vi "Dashboard Main.vi"() -> ()   [LabVIEW 2015]
uses:
  <vilib>/Utility/miscctls.llb/LVRowAndColumnTypeDef.ctl
  <vilib>/event_ctls.llb/eventvkey.ctl
  <vilib>/Rock Robotics/WPI/Dashboard/WPI_DashboardLogging Global.vi
  <vilib>/Rock Robotics/Network Tables/NT Read Numeric Array.vi
  <vilib>/Rock Robotics/Network Tables/NT Write String Array.vi
  <vilib>/Utility/config.llb/Write Key (String).vi
  <vilib>/Utility/config.llb/Write Key (I32).vi
  <vilib>/Utility/config.llb/NI_LVConfig.lvlib
panel:
  in  "TCP":refnum<k5>
  in  "Rec Mode":enum32{"Stop", "Record", "Playback"}(radio)
  in  "Vision":u16(ring) items=["Camera Off", "USB Camera SW", "USB Camera HW", "IP Camera"]
  out "Camera IP":string
  out "Image Message":string="Timeout in Camera Communications"
  in  "Dashboard Tab":T1(tab)
  in  "Select Auto":string(combo)
  out "NT Connection":bool
  in  "Camera Settings":T2={"Frame Rate"=30, "Compression"=30, "Size"=1} {"Frame Rate" scale=1.0..30.0; "Size" items=["640x480", "320x240", "160x120"]}
  out "MotorChart R":cluster{"Numeric":dbl, "Numeric":dbl}(graph)
  out "MotorChart L":T3(graph)
  out "MotorSliders R":cluster{"MotorSlide1":dbl, "MotorSlide2":dbl} {"MotorSlide2" scale=-1.0..1.0 scale format="%#_2e"; "MotorSlide1" scale=-1.0..1.0 scale format="%#_2e"}
  out "MotorSliders L":T4 {"MotorSlide4 2" scale=0.0..14.0 scale format="%#_2e"; "MotorSlide2" scale=-1.0..1.0 scale format="%#_2e"; "MotorSlide1" scale=-1.0..1.0 scale format="%#_2e"}
  out "JS1 Z":dbl(slide) scale=-1.0..1.0 scale format="%#_2e"
  out "JS1 Graph":cluster{"X":dbl, "Y":dbl}[](graph)
  out "JS1 Buttons":T5
  out "JS2 Z":dbl(slide) scale=-1.0..1.0 scale format="%#_2e"
  out "JS2 Graph":cluster{"X":dbl, "Y":dbl}[](graph)
  out "JS2 Buttons":T5
  out "Mode":T6(ring)=enum."Auto Disabled"
  in  "DB Camera Config":bool
  out "fps":dbl format="%#.1g"
  out "Mbps":dbl format="%#.1g"
  out "Mbps LED":bool
  in  "DB/String 9":string
  in  "DB/String 8":string
  in  "DB/String 7":string
  in  "DB/String 6":string
  in  "DB/String 5":string
  in  "DB/String 4":string
  in  "DB/String 3":string
  in  "DB/String 2":string
  in  "DB/String 1":string
  in  "DB/String 0":string
  in  "DB/Slider 0":dbl(slide) scale=0.0..5.0
  in  "DB/Slider 1":dbl(slide) scale=0.0..5.0
  in  "DB/Slider 2":dbl(slide) scale=0.0..5.0
  in  "DB/Slider 3":dbl(slide) scale=0.0..5.0
  out "DB/LED 3":bool
  out "DB/LED 2":bool
  out "DB/LED 1":bool
  out "DB/LED 0":bool
  in  "DB/Button 3":bool
  in  "DB/Button 2":bool
  in  "DB/Button 1":bool
  in  "DB/Button 0":bool caption="New Name"
  out "IMU AHRS":dbl[](array[numeric])
  out "CAN Current Values":dbl[](array[numeric])
  out "Arm Angle":dbl
  out "Right LIDAR":dbl
  out "Left LIDAR":dbl
  out "Right Encoder":dbl
  out "Left Encoder":dbl
  out "Ultrasonic Sensors":dbl[](array[numeric])
  out "SPI Gyro":dbl
  out "IMU AHRS Delta":dbl[](array[numeric])
  out "Goal Position":string
  out "appended array":string[](array[string])
  out "Position":i32
  out "Numeric":i32
  in  "Test Slider":dbl(slide) scale=0.0..100.0 scale format="%#_3g"
  in  "On/Off":bool caption="Solenoid"
  in  "Test Name":u16(ring) items=["Select the test to run..."]
  in  "Test Tree":string(tree)
  in  "Motor":cluster{"Value":dbl, "Enable":bool} {"Value" scale=-1.0..1.0 scale format="%#_3g"}
  out "Progress":T7 {"Test Progress" scale=0.0..100.0}
  in  "Rev/Fwd":cluster{"Forward":bool, "Reverse":bool}
  in  "Test Ring":u16(ring) items=["Monochrome", "Color"]
  out "Cmd Status":string
  in  "Execute Command":bool
  in  "Command Params":string[][](table)
  in  "Command Selection":i32(listbox)
  in  "Defence 5":bool
  in  "Defence 4":bool
  in  "Defence 3":bool
  in  "Defence 2":bool
  in  "Defence 1":bool
  in  "Defense 5":u16(ring)=8 items=["", "Portcullis", "Chili Fries", "Moat", "Ramparts", "Drawbridge", "Sally Port", "Rock Wall", "Rough Terrain"]
  in  "Defense 2":u16(ring)=8 items=["", "Portcullis", "Chili Fries", "Moat", "Ramparts", "Drawbridge", "Sally Port", "Rock Wall", "Rough Terrain"]
  in  "Defense 3":u16(ring)=8 items=["", "Portcullis", "Chili Fries", "Moat", "Ramparts", "Drawbridge", "Sally Port", "Rock Wall", "Rough Terrain"]
  in  "Defense 4":u16(ring)=8 items=["", "Portcullis", "Chili Fries", "Moat", "Ramparts", "Drawbridge", "Sally Port", "Rock Wall", "Rough Terrain"]
  in  "Defense 1":string="Low Bar"
  out "Robot":bool
  in  "Goal Position 3":u16(ring)=8 items=["", "Left", "Center", "Right"]
  in  "Goal Position 2":u16(ring)=8 items=["", "High", "Low"]
  in  "CheckList":i32(listbox)
  out "Tree":string(tree)
  out "Camera Image":T8(plugin-control)
  out "Background":bool
  # "Left"
  # "Front"
  # "Right"
  # "Battery"
  # "Pitch"
  # "Roll"
  # "Yaw"
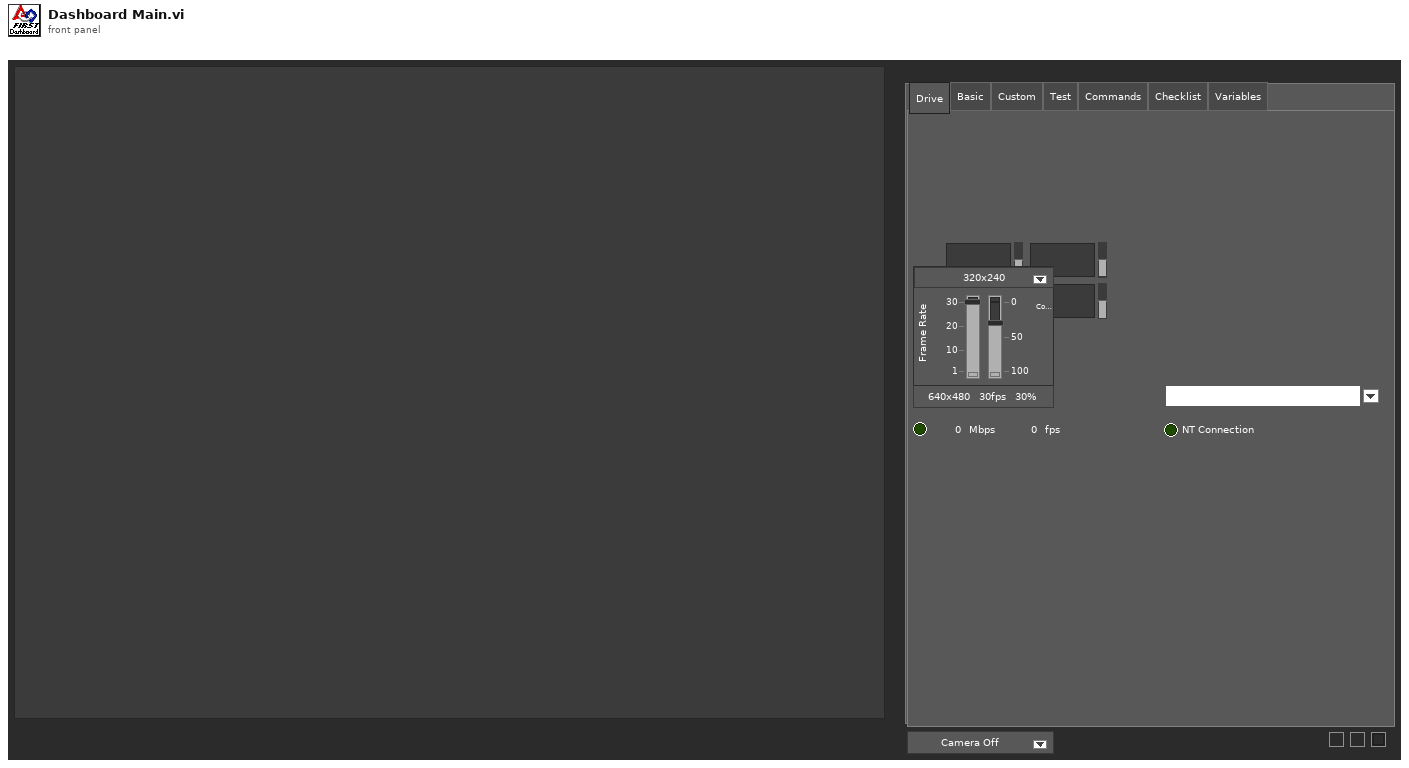
[diagram p1: front panel]
types:
  T1 = enum32{"Drive", "Basic", "Custom", "Test", "Commands", "Checklist", "Variables"}
  T2 = cluster{"Frame Rate":i32, "Compression":i32, "Size":u16}
  T3 = cluster{"Numeric":dbl, "Numeric":dbl, "Battery V":dbl}
  T4 = cluster{"MotorSlide1":dbl, "MotorSlide2":dbl, "MotorSlide4 2":dbl}
  T5 = cluster{bool, bool, bool, bool, bool, bool, bool, bool, bool, bool, bool, bool}
  T6 = enum8{"Tele-Op Disabled", "Tele-Op Enabled", "Auto Disabled", "Auto Enabled", "Test Disabled", "Test Enabled", "Disconnected", "No Code", "E-Stop"}
  T7 = cluster{"Test Progress":u8, "Test Progress Text":string}
  T8 = typedef "IMAQ Image.ctl" = refnum<image>
  T9 = cluster{"IDs":cluster{"RPC field ID":u16, "Unique ID":u16}, "String":string}
  T10 = enum32{"Drive", "Basic", "Custom", "Test", "Checklist", "Variables"}
  T11 = typedef "Image Type" = u32
  T12 = cluster{"Camera Image":refnum<vi>, "Dashboard Tab":refnum<vi>, "Background":refnum<vi>, "Vision":refnum<vi>, "Rec Mode":refnum<vi>, "Test Slider":refnum<vi>, "On/Off ":refnum<vi>, "Test Ring":refnum<vi>, "Rev/Fwd":refnum<vi>, "Test Name":refnum<vi>, "Motor":refnum<vi>, "Progress":refnum<vi>, "CheckList":refnum<vi>, "Tree":refnum<vi>, "Test Tree":refnum<vi>, "Command Params":refnum<vi>, "Command Selection":refnum<vi>, "Execute Command":refnum<vi>, "Cmd Status":refnum<vi>}
  T13 = cluster{"Error Strings":string, "Disable Counts":cluster{u16, u16}, "Rail Faults":cluster{u16, u16, u16}, "Robot IP":string, "DB Mode":u8, "Event Info":cluster{"Name":string, "Type":u8, "Number":u16, "Replay":u8}, "Camera Addr":string}
  T14 = cluster{"Storage":cluster{"Disk Free":u64, "RAM Block":u32, "RAM free":u32}, "CPU Utilization":cluster{"CPU % ISR":sgl, "CPU % Time Crit":sgl, "CPU % Timed Str":sgl, "CPU % High":sgl, "CPU % Above":sgl, "CPU % Normal":sgl, "CPU % Low":sgl}, "CAN":cluster{"% Bus Utilization":sgl, "Bus Off Cnt":u32, "TX_FIFO Full Cnt":u32, "Receive Error Cnt":u8, "Transmit Error Cnt":u8}, "HID":cluster{"HID Outputs":u32, "Rumble Low":u16, "Rumble High":u16}[]}
  T15 = cluster{"Status bits":cluster{"Test Mode":bool, "Autonomous":bool, "Enabled":bool, "Code Start":bool, "Brownout":bool, "Reserved 2":bool, "Reserved 3":bool, "E-Stop":bool}, "Code Trace":cluster{"Disabled":bool, "TeleOp":bool, "Auto":bool, "Test":bool}, "Controller Type":enum16{"unknown", "cRIO", "roboRio"}, "Code?":enum16{"unknown", "noCode", "code"}, "Battery V":dbl}
  T16 = cluster{"Control Bits":cluster{"TestMode":bool, "Autonomous":bool, "Enabled":bool, "FMS Present":bool, bool, bool, bool, "E-Stop":bool}, "Team Station ":u8, "Countdown":sgl, "Joystick Values":cluster{"Axes":dbl[], "Buttons":bool[], "POVs":i16[]}[]}
  T17 = cluster{"Axes":dbl[], "Buttons":bool[], "POVs":i16[]}[]
  T18 = cluster{"Axes":dbl[], "Buttons":bool[], "POVs":i16[]}
  T19 = cluster{"Buttons[0]":bool, "Buttons[1]":bool, "Buttons[2]":bool, "Buttons[3]":bool, "Buttons[4]":bool, "Buttons[5]":bool, "Buttons[6]":bool, "Buttons[7]":bool, "Buttons[8]":bool, "Buttons[9]":bool, "Buttons[10]":bool, "Buttons[11]":bool}
  T20 = typedef "NI_LVConfig.lvlib/Config Data RefNum.ctl" = refnum<k1>
  T21 = cluster{"Operation":enum16{"Update", "Clear"}, "Color Box":u32}[]
  T22 = typedef "eventvkey.ctl" = enum16{"ASCII", "Enter", "Return", "Shift", "Ctrl", "Alt", "Cmd", "Opt", "Caps", "NumLock", "Clear", "Break", "Up", "Down", "Left", "Right", "Insert", "Delete", "Home", "End", "PageUp", "PageDown", "Escape", "Help", "Pause", "ScrollLock", "F1", "F2", "F3", "F4", "F5", "F6", "F7", "F8", "F9", "F10", "F11", "F12", "F13", "F14", "F15", "F16", "F17", "F18", "F19", "F20", "F21", "F22", "F23", "F24", "Play", "VolumeUp", "VolumeDown", "Mute", "Two Byte Char"}
  T23 = cluster{"Image Size":bool, "Image Type":bool, "Pixel Value":bool, "ROI Information":bool, "Zoom Factor":bool}
  T24 = enum8{"Enabled", "Disabled", "Disabled and Grayed Out"}
  T25 = cluster{"Operation":enum16{"Update", "Clear"}, "Color Box":u32}
  T26 = typedef "LVRowAndColumnTypeDef.ctl" = cluster{"Row":i32, "Column":i32}
  T27 = cluster{"Shift":bool, "Ctrl":bool, "Alt":bool, "Cmd":bool, "Opt":bool}
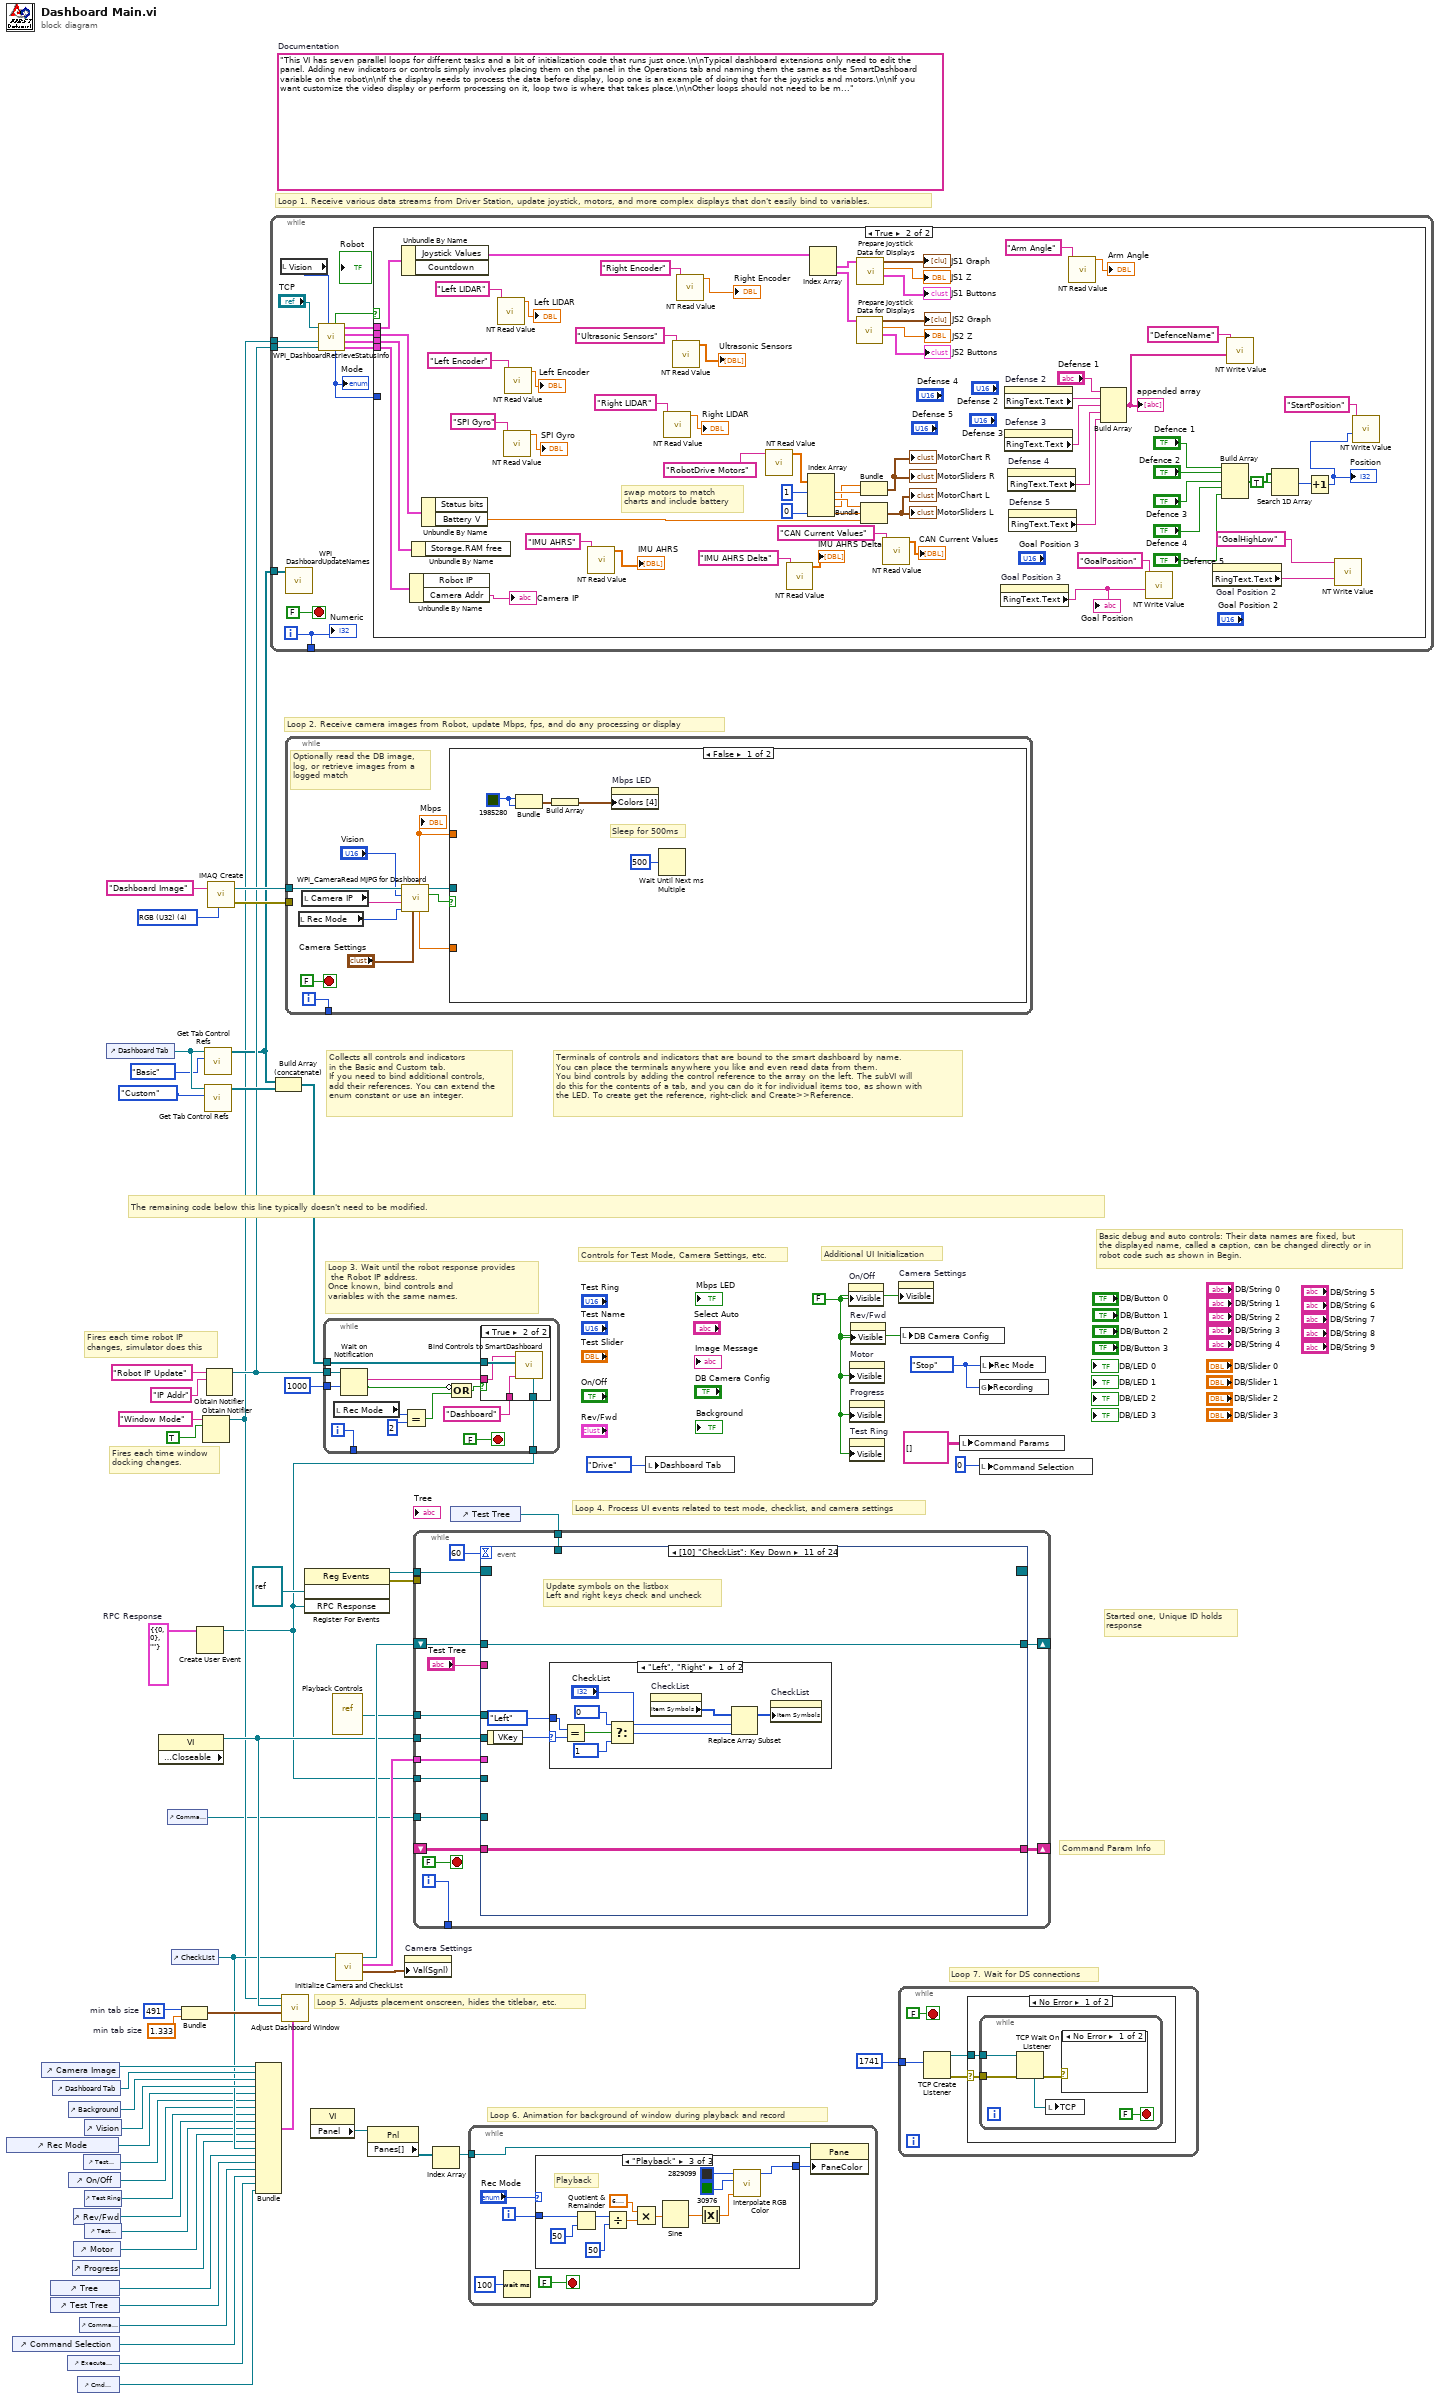
[diagram p0: block diagram]
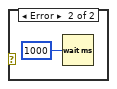
[diagram p2: hidden frame]
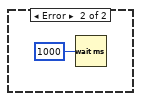
[diagram p3: hidden frame]
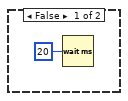
[diagram p4: hidden frame]
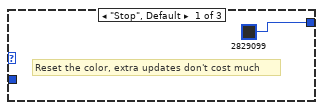
[diagram p5: hidden frame]
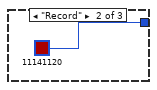
[diagram p6: hidden frame]
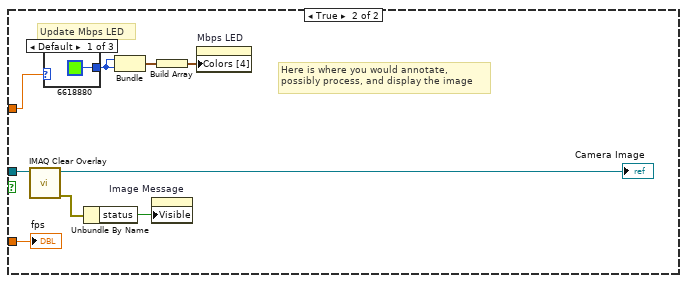
[diagram p8: hidden frame]
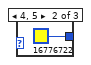
[diagram p9: hidden frame]
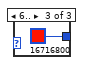
[diagram p10: hidden frame]
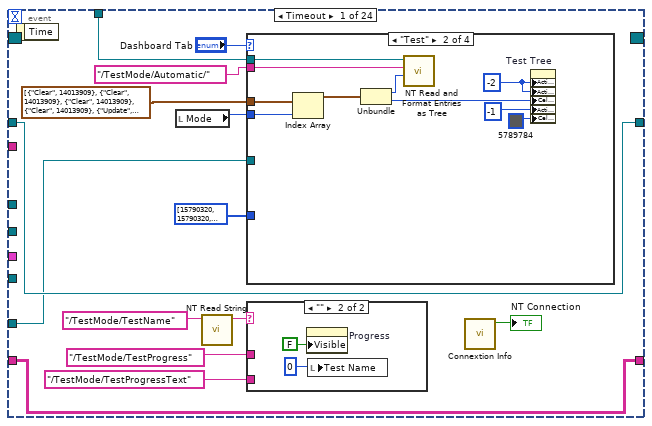
[diagram p11: hidden frame]
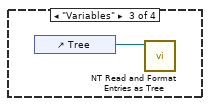
[diagram p13: hidden frame]
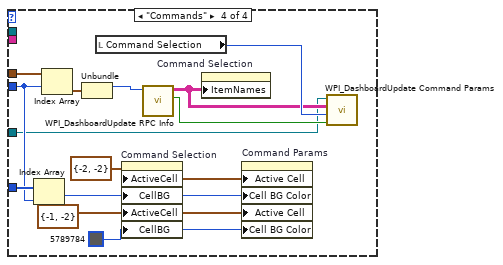
[diagram p14: hidden frame]
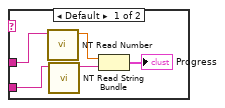
[diagram p15: hidden frame]
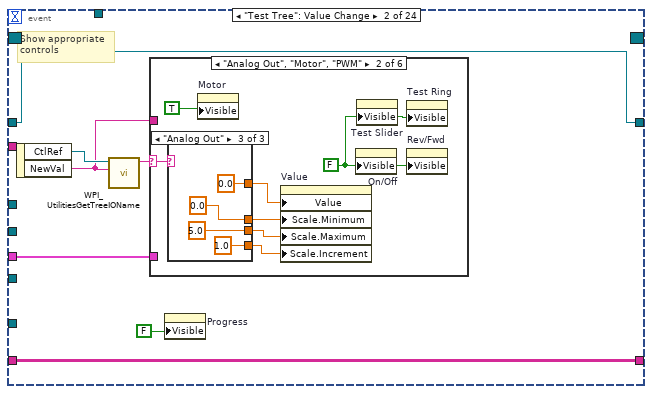
[diagram p16: hidden frame]
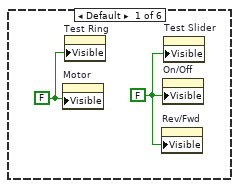
[diagram p17: hidden frame]
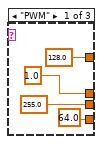
[diagram p18: hidden frame]
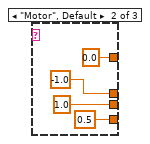
[diagram p19: hidden frame]
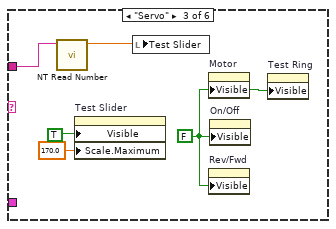
[diagram p20: hidden frame]
diagram:
  w7 = T9 {"IDs"={"RPC field ID"=0, "Unique ID"=0}, "String"=""}  # RPC Response
  w33 = 491  # min tab size
  w32 = 1.333  # min tab size
  w41 = enum32{"Stop", "Record", "Playback"}."Stop" ("Rec Mode")
  w15 = FALSE ("Visible")
  (unwired) "This VI has seven parallel loops for different tasks and a bit of initialization code that runs just once.\n\nTypical dashboard extensions only need to edit the panel. Adding new indicators or controls simply involves placing them on the panel in the Operations tab and naming them the same as the SmartDashboard variable on the robot\n\nIf the display needs to process the data before display, loop one is an example of doing that for the joysticks and motors.\n\nIf you want customize the video display or perform processing on it, loop two is where that takes place.\n\nOther loops should not need to be modified. They are pretty standard, and document the task they perform."  # Documentation
  w61 = T11 4 items=["Grayscale (U8)", "Grayscale (I16)", "Grayscale (SGL)", "Complex (CSG)", "RGB (U32)", "HSL (U32)", "RGB (U64)"] ("Image Type")
  # "Command Param Info"
  # "Started one, Unique ID holds\nresponse"
  # "Loop 7. Wait for DS connections"
  # "Basic debug and auto controls: Their data names are fixed, but\nthe displayed name, called a caption, can be changed directly or in\nrobot code such as shown in Begin."
  # "Controls for Test Mode, Camera Settings, etc."
  # "Additional UI Initialization"
  # "Loop 6. Animation for background of window during playback and record"
  # "Fires each time robot IP\nchanges, simulator does this"
  # "Fires each time window\ndocking changes."
  # "Collects all controls and indicators\nin the Basic and Custom tab.\nIf you need to bind additional controls,\nadd their references. You can extend the\nenum constant or use an integer."
  # "The remaining code below this line typically doesn't need to be modified."
  # "Loop 4. Process UI events related to test mode, checklist, and camera settings"
  # "Terminals of controls and indicators that are bound to the smart dashboard by name.\nYou can place the terminals anywhere you like and even read data from them.\nYou bind controls by adding the control reference to the array on the left. The subVI will\ndo this for the contents of a tab, and you can do it for individual items too, as shown with\nthe LED. To create get the reference, right-click and Create>>Reference."
  # "Loop 3. Wait until the robot response provides\n the Robot IP address.\nOnce known, bind controls and\nvariables with the same names."
  # "Loop 5. Adjusts placement onscreen, hides the titlebar, etc."
  # "Loop 1. Receive various data streams from Driver Station, update joystick, motors, and more complex displays that don't easily bind to variables."
  # "Loop 2. Receive camera images from Robot, update Mbps, fps, and do any processing or display"
  n1 = control-ref of="Rec Mode"() -> (w21:refnum<vi>)
  n2 = control-ref of="Command Selection"() -> (w6:refnum<vi>)
  n3 = control-ref of="Camera Image"() -> (w36:refnum<vi>)
  n4 = control-ref of="Tree"() -> (w25:refnum<vi>)
  n5 = control-ref of="Test Tree"() -> (w24:refnum<vi>)
  n6 = control-ref of="Dashboard Tab"() -> (w35:refnum<vi>)
  n7 = control-ref of="Execute Command"() -> (w8:refnum<vi>)
  n8 = control-ref of="Background"() -> (w30:refnum<vi>)
  n9 = control-ref of="On/Off"() -> (w19:refnum<vi>)
  n10 = control-ref of="Progress"() -> (w16:refnum<vi>)
  n11 = control-ref of="Rev/Fwd"() -> (w17:refnum<vi>)
  n12 = control-ref of="Motor"() -> (w22:refnum<vi>)
  n13 = control-ref of="Cmd Status"() -> (w2:refnum<vi>)
  n14 = control-ref of="Command Params"() -> (w9:refnum<vi>)
  n15 = control-ref of="Test Slider"() -> (w20:refnum<vi>)
  n16 = control-ref of="Vision"() -> (w34:refnum<vi>)
  n17 = control-ref of="Test Ring"() -> (w18:refnum<vi>)
  n18 = control-ref of="Test Name"() -> (w23:refnum<vi>)
  n19 = control-ref of="Dashboard Tab"() -> (w39:refnum<vi>)
  n20 = property class="VI" props=["Front Panel.Closeable"]() -> (reference out=w40:refnum<vi>)  [unwired: 2 in, 2 out]
  n21 = control-ref of="Command Params"() -> (w1:refnum<vi>)
  n22 = control-ref of="CheckList"() -> (w26:refnum<vi>)
  n23 = Bundle("min tab size"=w33, "min tab size"=w32) -> (w31:cluster{"min tab size":i32, "min tab size":dbl})  [unwired: 1 in]
  n24 = Create User Event(user event datatype=w7) -> (user event=w3:refnum<user-event>)  [unwired: 1 in, 1 out]
  n25 = Obtain Notifier(name (unnamed)="Window Mode", notification data type=TRUE) -> (notifier out=w12:refnum<notifier>)  [unwired: 2 in, 2 out]
  n26 = call <vilib>:"Get Tab Control Refs.vi"("Page Index"=T10."Basic" ("Dashboard Tab"), "TabControl in"=w39) -> ("ControlsOnPage"=w13:refnum<vi>[])  [unwired: 9 in]
  n27 = call <vilib>:"Get Tab Control Refs.vi"("Page Index"=T10."Custom" ("Dashboard Tab"), "TabControl in"=w39) -> ("ControlsOnPage"=w38:refnum<vi>[])  [unwired: 9 in]
  n28 = Obtain Notifier(name (unnamed)="Robot IP Update", notification data type="IP Addr" ("name (unnamed)")) -> (notifier out=w14:refnum<notifier>)  [unwired: 2 in, 2 out]
  n29 = call "IMAQ Create"("Image Name"="Dashboard Image", "Image Type"=w61) -> ("New Image"=w59:T8, "error out"=w58:errorcluster)  [unwired: 2 in, 1 out]
  n30 = Bundle("Camera Image"=w36, "Dashboard Tab"=w35, "Background"=w30, "Vision"=w34, "Rec Mode"=w21, "Test Slider"=w20, "On/Off"=w19, "Test Ring"=w18, "Rev/Fwd"=w17, "Test Name"=w23, "Motor"=w22, "Progress"=w16, "CheckList"=w26, "Tree"=w25, "Test Tree"=w24, "Command Params"=w9, "Command Selection"=w6, "Execute Command"=w8, "Cmd Status"=w2) -> (w27:T12)  [unwired: 1 in]
  n31 = while {
    tunnel: [w73] -> _
    tunnel: w14 -> [w67]
    tunnel: w13 -> [w66]
    tunnel: w12 -> [w62]
    i -> [w73]
    stop <- FALSE stop-if-true
    n32 = local read "Vision"() -> (w64:u16)
    n33 = call <vilib>:"WPI_DashboardUpdateNames.vi"("Controls on Tab"=w66) -> ()  [unwired: 11 in]
    n34 = call <vilib>:"WPI_DashboardRetrieveStatusInfo.vi"("Vision"=w64, "Binding Refnum"=w67, "Window Mode Notifier"=w62, "TCP Cnx"="TCP") -> ("Power and Errors"=w68:T13, "Robot Metrics"=w71:T14, "Status Info"=w72:T15, "Control Info"=w69:T16, "Robot Mode"=w65:T6, "Process?"=w70:bool)  [unwired: 2 in]
    "Mode" <- w65
    n35 = case shown="True" w70 {
      tunnel: w72 -> [_ w141]
      tunnel: w71 -> [_ w140]
      tunnel: w69 -> [_ w139]
      tunnel: w68 -> [_ w138]
      tunnel: w65 -> [_ _]
      frame False {
        n36 = Wait (ms)(milliseconds to wait=u32 20) -> ()  [unwired: 1 out]
      }
      frame True {
        # "swap motors to match\ncharts and include battery"
        n37 = Unbundle By Name(w139) -> ("Joystick Values"=w128:T17)  [unwired: 1 out]
        n38 = Unbundle By Name(w138) -> ("Camera Addr"=→"Camera IP":string)  [unwired: 1 out]
        n39 = Unbundle By Name(w140) -> ()  [unwired: 1 out]
        n40 = Unbundle By Name(w141) -> ("Battery V"=w129:dbl)  [unwired: 1 out]
        n41 = call-poly <vilib>:"NT Read Value.vi"("Name"="Left LIDAR") -> ("Numeric"=→"Left LIDAR":dbl)  [unwired: 9 in, 1 out]
        n42 = call-poly <vilib>:"NT Read Value.vi"("Name"="SPI Gyro") -> ("Numeric"=→"SPI Gyro":dbl)  [unwired: 9 in, 1 out]
        n43 = call-poly <vilib>:"NT Read Value.vi"("Name"="Left Encoder") -> ("Numeric"=→"Left Encoder":dbl)  [unwired: 9 in, 1 out]
        n44 = call-poly <vilib>:"NT Read Value.vi"("Name"="IMU AHRS") -> ("Numeric Array"=→"IMU AHRS":dbl[])  [unwired: 9 in, 1 out]
        n45 = call-poly <vilib>:"NT Read Value.vi"("Name"="Right LIDAR") -> ("Numeric"=→"Right LIDAR":dbl)  [unwired: 9 in, 1 out]
        n46 = call-poly <vilib>:"NT Read Value.vi"("Name"="Ultrasonic Sensors") -> ("Numeric Array"=→"Ultrasonic Sensors":dbl[])  [unwired: 9 in, 1 out]
        n47 = call-poly <vilib>:"NT Read Value.vi"("Name"="Right Encoder") -> ("Numeric"=→"Right Encoder":dbl)  [unwired: 9 in, 1 out]
        n48 = call-poly <vilib>:"NT Read Value.vi"("Name"="RobotDrive Motors") -> ("Numeric Array"=w117:dbl[])  [unwired: 9 in, 1 out]
        n49 = call-poly <vilib>:"NT Read Value.vi"("Name"="IMU AHRS Delta") -> ("Numeric Array"=→"IMU AHRS Delta":dbl[])  [unwired: 9 in, 1 out]
        n50 = Index Array(array=w117, index #1=1, index #4=0) -> (element #1=w133:dbl, element #2=w134:dbl, element #3=w132:dbl, element #4=w137:dbl)  [unwired: 2 in]
        n51 = Index Array(array=w128) -> (element #1=w127:T18, element #2=w122:T18)  [unwired: 2 in]
        n52 = call "Prepare Joystick Data for Displays.vi"("Joystick Values"=w122) -> ("Buttons"=→"JS2 Buttons":T19, "Z Axis"=→"JS2 Z":dbl, "Cartesian Data"=→"JS2 Graph":cluster{"X axis":dbl, "X axis":dbl}[])  [unwired: 8 in]
        n53 = call "Prepare Joystick Data for Displays.vi"("Joystick Values"=w127) -> ("Buttons"=→"JS1 Buttons":T19, "Z Axis"=→"JS1 Z":dbl, "Cartesian Data"=→"JS1 Graph":cluster{"X axis":dbl, "X axis":dbl}[])  [unwired: 8 in]
        n54 = Bundle("Numeric"=w132, "Numeric"=w133) -> (→"MotorChart R" →"MotorSliders R":cluster{"Numeric":dbl, "Numeric":dbl})  [unwired: 1 in]
        n55 = Bundle("Numeric"=w134, "Numeric"=w137, "Battery V"=w129) -> (→"MotorChart L" →"MotorSliders L":T3)  [unwired: 1 in]
        n56 = call-poly <vilib>:"NT Read Value.vi"("Name"="CAN Current Values") -> ("Numeric Array"=→"CAN Current Values":dbl[])  [unwired: 9 in, 1 out]
        n57 = property on="Goal Position 3" class="Ring (strict)"() -> ("RingText.Text"=w88:string)  [unwired: 2 in, 2 out]
        "Goal Position" <- w88
        n58 = property on="Defense 2" class="Ring (strict)"() -> ("RingText.Text"=w95:string)  [unwired: 2 in, 2 out]
        n59 = property on="Defense 3" class="Ring (strict)"() -> ("RingText.Text"=w94:string)  [unwired: 2 in, 2 out]
        n60 = property on="Defense 4" class="Ring (strict)"() -> ("RingText.Text"=w93:string)  [unwired: 2 in, 2 out]
        n61 = property on="Defense 5" class="Ring (strict)"() -> ("RingText.Text"=w92:string)  [unwired: 2 in, 2 out]
        n62 = call-poly <vilib>:"NT Read Value.vi"("Name"="Arm Angle") -> ("Numeric"=→"Arm Angle":dbl)  [unwired: 9 in, 1 out]
        n63 = Build Array("Defense 1", w95, w94, w93, w92) -> (w90:string[])
        "appended array" <- w90
        n64 = call-poly <vilib>:"NT Write Value.vi"("String"=w88, "Name"="GoalPosition") -> ()  [unwired: 9 in, 1 out]
        n65 = property on="Goal Position 2" class="Ring (strict)"() -> ("RingText.Text"=w76:string)  [unwired: 2 in, 2 out]
        n66 = Build Array("Defence 1", "Defence 2", "Defence 3", "Defence 4", "Defence 5") -> (w85:bool[])
        n67 = call-poly <vilib>:"NT Write Value.vi"("String Array"=w90, "Name"="DefenceName") -> ()  [unwired: 9 in, 1 out]
        n68 = Search 1D Array(1D array=w85, element=TRUE) -> (index of element=w87:i32)  [unwired: 1 in]
        n69 = Increment(x=w87) -> (x+1=w78:i32)
        "Position" <- w78
        n70 = call-poly <vilib>:"NT Write Value.vi"("String"=w76, "Name"="GoalHighLow") -> ()  [unwired: 9 in, 1 out]
        n71 = call-poly <vilib>:"NT Write Value.vi"("Numeric"=w78, "Name"="StartPosition") -> ()  [unwired: 9 in, 1 out]
      }
    }
    "Numeric" <- w73
  }
  n72 = Build Array (concatenate)(w13, w38) -> (w37:refnum<vi>[])
  n73 = call "Adjust Dashboard Window.vi"("Sizing Refnums"=w27, "Size Constraints"=w31, "VI"=w40, "WIn Mode"=w12) -> ()  [unwired: 8 in]
  n74 = while {
    tunnel: w59 -> [w150]
    tunnel: w58 -> [_]
    tunnel: [w151] -> _
    i -> [w151]
    stop <- FALSE stop-if-true
    # "Optionally read the DB image,\nlog, or retrieve images from a\nlogged match"
    n75 = local read "Rec Mode"() -> (w145:enum32{"Stop", "Record", "Playback"})
    n76 = local read "Camera IP"() -> (w143:string)
    n77 = call <vilib>:"WPI_CameraRead MJPG for Dashboard.vi"("Camera Settings"="Camera Settings", "Rec Mode"=w145, "Camera IP"=w143, "Camera Mode"="Vision", "Refnum in"=w150) -> ("Active"=w148:bool, "Refnum out"=w149:T8, "FPS"=w147:dbl, "Bandwidth (Mbps)"=w142:dbl)  [unwired: 3 in]
    "Mbps" <- w142
    n78 = case shown="False" w148 {
      tunnel: w149 -> [_ w160]
      tunnel: w142 -> [_ w159]
      tunnel: w147 -> [_ w157]
      frame False {
        w153 = u32 1985280 ("Color Box")
        # "Sleep for 500ms"
        n79 = Bundle("Color Box"=w153, "Color Box"=w153) -> (w155:cluster{"Color Box":u32, "Color Box":u32})  [unwired: 1 out]
        n80 = Build Array(w155) -> (w154:cluster{"Color Box":u32, "Color Box":u32}[])
        n81 = property on="Mbps LED" class="Bool (strict)"("Colors [4]"=w154) -> ()  [unwired: 2 in, 2 out]
        n82 = Wait Until Next ms Multiple(millisecond multiple=u32 500) -> ()  [unwired: 1 out]
      }
      frame True {
        # "Here is where you would annotate,\npossibly process, and display the image"
        # "Update Mbps LED"
        n83 = call "IMAQ Clear Overlay"("Image"=w160) -> ("error out"=w164:errorcluster, "Image Out"=→"Camera Image":T8)  [unwired: 2 in, 7 out]
        n84 = case shown="Default" w159 {
          tunnel: [u32 6618880 ("Color Box") u32 16776722 ("Color Box") u32 16716800 ("Color Box")] -> w161
          frame Default {
          }
          frame 4, 5 {
          }
          frame 6.. {
          }
        }
        n85 = Unbundle By Name(w164) -> ("status"=w165:bool)
        n86 = Bundle("Color Box"=w161, "Color Box"=w161) -> (w163:cluster{"Color Box":u32, "Color Box":u32})  [unwired: 1 out]
        n87 = property on="Image Message" class="Str"("Visible"=w165) -> ()  [unwired: 2 in, 2 out]
        n88 = Build Array(w163) -> (w162:cluster{"Color Box":u32, "Color Box":u32}[])
        n89 = property on="Mbps LED" class="Bool (strict)"("Colors [4]"=w162) -> ()  [unwired: 2 in, 2 out]
        "fps" <- w157
      }
    }
  }
  n90 = register-events(refnum<vi> refnum, w3) -> (reference out=w45:refnum<event-registration>, error out=w44:errorcluster)  [unwired: 2 in]
  n91 = property class="VI"() -> ("Panel"=w48:refnum<vi>)  [unwired: 2 in, 2 out]
  n92 = while {
    tunnel: w37 -> [w181]
    tunnel: w14 -> [w179]
    tunnel: [w177] -> _
    tunnel: u32 1000 ("milliseconds to wait") -> [w176]
    tunnel: w3 -> [w169]
    i -> [w177]
    stop <- FALSE stop-if-true
    n93 = local read "Rec Mode"() -> (w172:enum32{"Stop", "Record", "Playback"})
    n94 = Wait on Notification(notifier=w179, timeout in ms (-1)=w176) -> (notification=w178:string, timed out?=w174:bool)  [unwired: 2 in, 2 out]
    n95 = Equal?(x=w172, y=u16 2 ("Rec Mode")) -> (x = y?=w173:bool)
    n96 = Compound Arithmetic op=OR(invert w174, w173) -> (w175:bool)
    n97 = case shown="True" w175 {
      tunnel: w181 -> [_ w185]
      tunnel: w178 -> [_ w184]
      tunnel: "Dashboard" -> [_ w183]
      tunnel: w169 -> [_ w182]
      frame False {
      }
      frame True {
        n98 = call <vilib>:"Bind Controls to SmartDashboard.vi"("RPC ref"=w182, "Client Name"=w183, "Bound Control Refs"=w185, "Server IP Address"=w184) -> ()  [unwired: 8 in]
      }
    }
  }
  n99 = vi-ref "Playback Controls.vi"() -> (w46:refnum<vi>)
  n100 = call "Initialize Camera and CheckList.vi"("ListBox in"=w26) -> ("Cluster"=w52:cluster{"value":i32, "value":i32, "index":i32}, "Array"=w53:cluster{string[]}[], "File Refnum"=w51:T20)  [unwired: 8 in]
  n101 = property class="Pnl"(reference=w48) -> ("Panes[]"=w49:refnum<vi>[])  [unwired: 1 in, 2 out]
  n102 = property on="Camera Settings" class="Clust (strict)"("Val(Sgnl)"=w52) -> ()  [unwired: 2 in, 2 out]
  n103 = Index Array(array=w49) -> (element=w47:refnum<vi>)  [unwired: 1 in]
  n104 = control-ref of="Test Tree"() -> (w50:refnum<vi>)
  n105 = while {
    tunnel: w53 -> [w197]
    shift-right: [w196] -> _
    shift-left: w51 -> [w195]
    tunnel: [w194] -> _
    tunnel: w50 -> [w193]
    tunnel: w46 -> [w192]
    tunnel: w45 -> [w191]
    tunnel: w44 -> [_]
    tunnel: w40 -> [w190]
    tunnel: w3 -> [w189]
    tunnel: w1 -> [w188]
    shift-right: [w187] -> _
    shift-left: _ -> [w186]
    i -> [w194]
    stop <- FALSE stop-if-true
    n106 = event shown="[10] \"CheckList\": Key Down" {
      selector: w191 -> [_ _ _ _ _ _ _ _ _ _ _ _ _ _ _ _ _ _ _ _ _ _ _ _]
      dyn-events: [_ _ _ _ _ _ _ _ _ _ _ _ _ _ _ _ _ _ w506 _ _ _ _ _] -> _
      timeout: u32 60 ("milliseconds to wait") -> [_ _ _ _ _ _ _ _ _ _ _ _ _ _ _ _ _ _ _ _ _ _ _ _]
      tunnel: w193 -> [w210 _ _ _ _ _ _ _ _ _ _ _ _ _ _ _ _ _ _ _ _ _ _ _]
      tunnel: "Test Tree" -> [_ _ _ _ _ _ _ _ _ _ _ _ _ w469 w478 w481 w486 w495 _ _ _ _ _ _]
      tunnel: w197 -> [_ w248 _ _ _ _ _ _ _ _ _ w431 w462 _ _ _ _ _ _ _ _ _ _ _]
      tunnel: [w207 w247 w351 w357 w367 w371 w377 w389 w397 w403 w416 w430 w455 w468 w476 w480 w485 w494 w508 w524 w526 w534 w545 w550] -> w196
      tunnel: w195 -> [w207 w247 w351 w357 w367 w371 w377 w389 w397 w403 w416 w429 w455 w468 w476 w480 w485 w494 w508 w524 w526 w534 w545 w550]
      tunnel: w192 -> [_ _ _ _ _ _ _ _ _ _ _ _ _ _ _ _ _ _ w509 _ w529 _ _ _]
      tunnel: w190 -> [_ _ _ _ _ _ _ _ _ _ _ _ _ _ _ _ _ _ w504 _ _ _ _ _]
      tunnel: w189 -> [_ _ _ _ _ _ _ _ _ _ _ _ _ _ _ _ _ _ w500 _ _ _ _ _]
      tunnel: w188 -> [w202 _ _ _ _ _ w375 _ _ _ _ _ _ _ _ _ _ _ _ _ _ _ _ _]
      tunnel: [w201 w246 w350 w356 w366 w372 w373 w383 w394 w402 w415 w428 w454 w467 w475 w479 w484 w493 w499 w522 w525 w530 w538 w551] -> w187
      tunnel: w186 -> [w201 w246 w350 w356 w366 w372 w373 _ _ w402 w415 w428 w454 w467 w475 w479 w484 w493 w499 w522 w525 w530 w538 w551]
      event Timeout {
        n107 = event-data() -> ()  [unwired: 1 in, 1 out]
        n108 = local read "Mode"() -> (w204:T6)
        n109 = call <vilib>:"NT Read String.vi"("Name"="/TestMode/TestName") -> ("String"=w213:string)  [unwired: 9 in, 1 out]
        n110 = case shown="\"Test\"" "Dashboard Tab" {
          tunnel: w210 -> [_ w224 _ _]
          tunnel: "/TestMode/Automatic/" ("Name Pattern") -> [_ w223 _ _]
          tunnel: T21 [{"Operation"=enum."Clear", "Color Box"=14013909}, {"Operation"=enum."Clear", "Color Box"=14013909}, {"Operation"=enum."Clear", "Color Box"=14013909}, {"Operation"=enum."Clear", "Color Box"=14013909}, {"Operation"=enum."Update", "Color Box"=14013909}, {"Operation"=enum."Update", "Color Box"=16777215}, {"Operation"=enum."Clear", "Color Box"=14013909}, {"Operation"=enum."Clear", "Color Box"=14013909}, {"Operation"=enum."Clear", "Color Box"=14013909}] -> [_ w216 _ w233]
          tunnel: w204 -> [_ w215 _ w232]
          tunnel: u32[] [15790320, 15790320, 15790320, 15790320, 16777215, 16777215, 15790320, 15790320, 15790320] -> [_ _ _ w238]
          tunnel: w202 -> [_ _ _ w226]
          frame "Custom", Default {
          }
          frame "Test" {
            w222 = -2 ("Active Item:Row Number")
            n111 = Index Array(array=w216, index=w215) -> (element=w217:T25)
            n112 = Unbundle(w217) -> ("Operation"=w218:enum16{"Update", "Clear"}, "Color Box"=w219:u32)
            n113 = call <vilib>:"NT Read and Format Entries as Tree.vi"("Operation"=w218, "Name Pattern"=w223, "Tree Refnum"=w224) -> ()  [unwired: 7 in, 2 out]
            n114 = property on="Test Tree" class="Tree (strict)"("Active Item Row Number"=w222, "ActiveColNum"=w222, "CellBG"=w219, "Active Item Row Number"=-1 ("Active Item:Row Number"), "CellBG"=u32 5789784 ("Color Box")) -> ()  [unwired: 2 in, 2 out]
          }
          frame "Variables" {
            n115 = control-ref of="Tree"() -> (w225:refnum<vi>)
            n116 = call <vilib>:"NT Read and Format Entries as Tree.vi"("Tree Refnum"=w225) -> ()  [unwired: 9 in, 2 out]
          }
          frame "Commands" {
            w234 = u32 5789784 ("Color Box")
            w235 = T26 {"Row"=-1, "Column"=-2} ("Active Cell:Active Cell")
            w237 = T26 {"Row"=-2, "Column"=-2} ("Active Cell:Active Cell")
            n117 = Index Array(array=w238, index=w232) -> (element=w236:u32)
            n118 = Index Array(array=w233, index=w232) -> (element=w231:T25)
            n119 = Unbundle(w231) -> ("Operation"=w230:enum16{"Update", "Clear"})  [unwired: 1 out]
            n120 = local read "Command Selection"() -> (w229:i32)
            n121 = property on="Command Selection" class="MCListbox (strict)"("ActiveCell"=w237, "CellBG"=w236, "ActiveCell"=w235, "CellBG"=w234) -> ()  [unwired: 2 in, 2 out]
            n122 = call <vilib>:"WPI_DashboardUpdate RPC Info.vi"("Operation"=w230) -> ("update"=w228:bool, "commands"=w227:string[][])  [unwired: 9 in]
            n123 = property on="Command Selection" class="MCListbox (strict)"("ItemNames"=w227) -> ()  [unwired: 2 in, 2 out]
            n124 = property on="Command Params" class="Tbl (strict)"("Active Cell"=w237, "Cell BG Color"=w236, "Active Cell"=w235, "Cell BG Color"=w234) -> ()  [unwired: 2 in, 2 out]
            n125 = call <vilib>:"WPI_DashboardUpdate Command Params.vi"("Update"=w228, "NewVal"=w229, "Commands"=w227, "Param Tbl"=w226) -> ()  [unwired: 7 in, 1 out]
          }
        }
        n126 = case shown="\"\"" w213 {
          tunnel: "/TestMode/TestProgress" ("Name") -> [w240 _]
          tunnel: "/TestMode/TestProgressText" ("Name") -> [w239 _]
          frame Default {
            n127 = call <vilib>:"NT Read Number.vi"("Name"=w240) -> ("Numeric"=w241:dbl)  [unwired: 9 in, 1 out]
            n128 = call <vilib>:"NT Read String.vi"("Name"=w239) -> ("String"=w242:string)  [unwired: 9 in, 1 out]
            n129 = Bundle("Numeric"=w241, "String"=w242) -> (→"Progress":cluster{"Numeric":dbl, "String":string})  [unwired: 1 in]
          }
          frame "" {
            n130 = property on="Progress" class="Clust (strict)"("Visible"=FALSE) -> ()  [unwired: 2 in, 2 out]
            n131 = local write "Test Name"(u16 0) -> ()
          }
        }
        n132 = call <vilib>:"Connextion Info.vi"() -> ("Connected"=→"NT Connection":bool)  [unwired: 10 in, 1 out]
      }
      event "Test Tree": Value Change {
        # "Show appropriate\ncontrols"
        n133 = event-data() -> ("CtlRef"=w251:refnum<vi>, "NewVal"=w249:string)  [unwired: 1 in]
        n134 = call <vilib>:"WPI_UtilitiesGetTreeIOName.vi"("NewVal"=w249, "TreeControl in"=w251) -> ("I/O Name"=w252:string)  [unwired: 9 in]
        n135 = case shown="\"Analog Out\", \"Motor\", \"PWM\"" w252 {
          selector: w252 -> [_ w259 _ w281 w290 _]
          tunnel: w249 -> [_ _ w278 w280 _ w297]
          tunnel: w248 -> [_ _ _ _ _ w296]
          frame Default {
            w254 = FALSE ("Visible")
            w253 = FALSE ("Visible")
            n136 = property on="Motor" class="Clust (strict)"("Visible"=w253) -> ()  [unwired: 2 in, 2 out]
            n137 = property on="Test Ring" class="Ring (strict)"("Visible"=w253) -> ()  [unwired: 2 in, 2 out]
            n138 = property on="Rev/Fwd" class="Clust (strict)"("Visible"=w254) -> ()  [unwired: 2 in, 2 out]
            n139 = property on="On/Off" class="Bool (strict)"("Visible"=w254) -> ()  [unwired: 2 in, 2 out]
            n140 = property on="Test Slider" class="Slide (strict)"("Visible"=w254) -> ()  [unwired: 2 in, 2 out]
          }
          frame "Analog Out", "Motor", "PWM" {
            w260 = FALSE ("Visible")
            n141 = case shown="\"Analog Out\"" w259 {
              tunnel: [1.0 ("Value") -1.0 ("Value") 0.0 ("Value")] -> w258
              tunnel: [255.0 ("Value") 1.0 ("Value") 5.0 ("Value")] -> w257
              tunnel: [128.0 ("Value") 0.0 ("Value") 0.0 ("Value")] -> w256
              tunnel: [64.0 ("Value") 0.5 ("Value") 1.0 ("Value")] -> w255
              frame "PWM" {
              }
              frame "Motor", Default {
              }
              frame "Analog Out" {
              }
            }
            n142 = property on="Motor" class="Clust (strict)"("Visible"=TRUE) -> ()  [unwired: 2 in, 2 out]
            n143 = property on="Value" class="Slide (strict)"("Value"=w256, "Scale.Minimum"=w258, "Scale.Maximum"=w257, "Scale.Increment"=w255) -> ()  [unwired: 2 in, 2 out]
            n144 = property on="On/Off" class="Bool (strict)"("Visible"=w260) -> ()  [unwired: 2 in, 2 out]
            n145 = property on="Test Slider" class="Slide (strict)"("Visible"=w260) -> ()  [unwired: 2 in, 2 out]
            n146 = property on="Test Ring" class="Ring (strict)"("Visible"=w260) -> ()  [unwired: 2 in, 2 out]
            n147 = property on="Rev/Fwd" class="Clust (strict)"("Visible"=w260) -> ()  [unwired: 2 in, 2 out]
          }
          frame "Servo" {
            w276 = FALSE ("Visible")
            n148 = call <vilib>:"NT Read Number.vi"("Name"=w278) -> ("Numeric"=w277:dbl)  [unwired: 9 in, 1 out]
            n149 = property on="Test Slider" class="Slide (strict)"("Visible"=TRUE, "Scale.Maximum"=170.0 ("Scale.Range:Maximum")) -> ()  [unwired: 2 in, 2 out]
            n150 = local write "Test Slider"(w277) -> ()
            n151 = property on="Motor" class="Clust (strict)"("Visible"=w276) -> ()  [unwired: 2 in, 2 out]
            n152 = property on="Rev/Fwd" class="Clust (strict)"("Visible"=w276) -> ()  [unwired: 2 in, 2 out]
            n153 = property on="On/Off" class="Bool (strict)"("Visible"=w276) -> ()  [unwired: 2 in, 2 out]
            n154 = property on="Test Ring" class="Ring (strict)"("Visible"=w276) -> ()  [unwired: 2 in, 2 out]
          }
          frame "Relay", "Solenoid" {
            w279 = FALSE ("Visible")
            n155 = property on="Motor" class="Clust (strict)"("Visible"=w279) -> ()  [unwired: 2 in, 2 out]
            n156 = property on="Test Slider" class="Slide (strict)"("Visible"=w279) -> ()  [unwired: 2 in, 2 out]
            n157 = Search and Replace String(input string=w280, search string="/Value  **", replace string="/Direction") -> (result string=w286:string)  [unwired: 5 in, 3 out]
            n158 = property on="Test Ring" class="Ring (strict)"("Visible"=w279) -> ()  [unwired: 2 in, 2 out]
            n159 = call <vilib>:"NT Read String.vi"("Name"=w286) -> ("String"=w284:string)  [unwired: 9 in, 1 out]
            n160 = Equal?(x="Both directions", y=w284) -> (x = y?=w282:bool)
            n161 = Not(x=w282) -> (.not. x?=w283:bool)
            n162 = property on="Rev/Fwd" class="Clust (strict)"("Visible"=w282) -> ()  [unwired: 2 in, 2 out]
            n163 = property on="On/Off" class="Bool (strict)"("Visible"=w283, "Caption.Text"=w281) -> ()  [unwired: 2 in, 2 out]
          }
          frame "Compressor", "Digital Out" {
            w289 = FALSE ("Visible")
            # "Get direction and finish"
            n164 = property on="Motor" class="Clust (strict)"("Visible"=w289) -> ()  [unwired: 2 in, 2 out]
            n165 = property on="Test Slider" class="Slide (strict)"("Visible"=w289) -> ()  [unwired: 2 in, 2 out]
            n166 = property on="Test Ring" class="Ring (strict)"("Visible"=w289) -> ()  [unwired: 2 in, 2 out]
            n167 = property on="On/Off" class="Bool (strict)"("Visible"=TRUE, "Caption.Text"=w290) -> ()  [unwired: 2 in, 2 out]
            n168 = property on="Rev/Fwd" class="Clust (strict)"("Visible"=FALSE) -> ()  [unwired: 2 in, 2 out]
          }
          frame "Camera" {
            n169 = call <vilib>:"Get Last Path Segment.vi"("String in"=w297) -> ("String out"=w298:string)  [unwired: 10 in]
            n170 = property on="On/Off" class="Bool (strict)"("Visible"=FALSE) -> ()  [unwired: 2 in, 2 out]
            n171 = property on="Motor" class="Clust (strict)"("Visible"=FALSE) -> ()  [unwired: 2 in, 2 out]
            n172 = property on="Rev/Fwd" class="Clust (strict)"("Visible"=FALSE) -> ()  [unwired: 2 in, 2 out]
            n173 = case shown="\"White Balance  **\"" w298 {
              tunnel: w297 -> [w304 w313 w322 w331 w340 _ w346]
              tunnel: w296 -> [w302 w310 w319 w328 w337 _ _]
              frame "Size  **" {
                n174 = Index Array(array=w302) -> (element=w301:cluster{string[]})  [unwired: 1 in]
                n175 = call <vilib>:"NT Read String.vi"("Name"=w304) -> ("String"=w303:string)  [unwired: 9 in, 1 out]
                n176 = Unbundle(w301) -> (w299:string[])
                n177 = Match First String(2:w299, 3:w303) -> (0:w300:i32)  [unwired: 1 out]
                n178 = property on="Test Ring" class="Ring (strict)"("Value"=w300, "Strings []"=w299) -> ()  [unwired: 2 in, 2 out]
                n179 = property on="Test Ring" class="Ring (strict)"("Visible"=TRUE) -> ()  [unwired: 2 in, 2 out]
                n180 = property on="Test Slider" class="Slide (strict)"("Visible"=FALSE) -> ()  [unwired: 2 in, 2 out]
              }
              frame "White Balance  **" {
                n181 = Index Array(array=w310, index=1) -> (element=w311:cluster{string[]})
                n182 = call <vilib>:"NT Read String.vi"("Name"=w313) -> ("String"=w312:string)  [unwired: 9 in, 1 out]
                n183 = Unbundle(w311) -> (w308:string[])
                n184 = Match First String(2:w308, 3:w312) -> (0:w307:i32)  [unwired: 1 out]
                n185 = property on="Test Ring" class="Ring (strict)"("Value"=w307, "Strings []"=w308) -> ()  [unwired: 2 in, 2 out]
                n186 = property on="Test Ring" class="Ring (strict)"("Visible"=TRUE) -> ()  [unwired: 2 in, 2 out]
                n187 = property on="Test Slider" class="Slide (strict)"("Visible"=FALSE) -> ()  [unwired: 2 in, 2 out]
              }
              frame "Exposure  **" {
                n188 = Index Array(array=w319, index=2) -> (element=w320:cluster{string[]})
                n189 = call <vilib>:"NT Read String.vi"("Name"=w322) -> ("String"=w321:string)  [unwired: 9 in, 1 out]
                n190 = Unbundle(w320) -> (w316:string[])
                n191 = Match First String(2:w316, 3:w321) -> (0:w317:i32)  [unwired: 1 out]
                n192 = property on="Test Ring" class="Ring (strict)"("Value"=w317, "Strings []"=w316) -> ()  [unwired: 2 in, 2 out]
                n193 = property on="Test Ring" class="Ring (strict)"("Visible"=TRUE) -> ()  [unwired: 2 in, 2 out]
                n194 = property on="Test Slider" class="Slide (strict)"("Visible"=FALSE) -> ()  [unwired: 2 in, 2 out]
              }
              frame "Exposure Priority  **" {
                n195 = Index Array(array=w328, index=3) -> (element=w329:cluster{string[]})
                n196 = call <vilib>:"NT Read String.vi"("Name"=w331) -> ("String"=w330:string)  [unwired: 9 in, 1 out]
                n197 = Unbundle(w329) -> (w325:string[])
                n198 = Match First String(2:w325, 3:w330) -> (0:w326:i32)  [unwired: 1 out]
                n199 = property on="Test Ring" class="Ring (strict)"("Value"=w326, "Strings []"=w325) -> ()  [unwired: 2 in, 2 out]
                n200 = property on="Test Ring" class="Ring (strict)"("Visible"=TRUE) -> ()  [unwired: 2 in, 2 out]
                n201 = property on="Test Slider" class="Slide (strict)"("Visible"=FALSE) -> ()  [unwired: 2 in, 2 out]
              }
              frame "Color Enable  **" {
                n202 = Index Array(array=w337, index=4) -> (element=w338:cluster{string[]})
                n203 = call <vilib>:"NT Read String.vi"("Name"=w340) -> ("String"=w339:string)  [unwired: 9 in, 1 out]
                n204 = Unbundle(w338) -> (w334:string[])
                n205 = Match First String(2:w334, 3:w339) -> (0:w335:i32)  [unwired: 1 out]
                n206 = property on="Test Ring" class="Ring (strict)"("Value"=w335, "Strings []"=w334) -> ()  [unwired: 2 in, 2 out]
                n207 = property on="Test Ring" class="Ring (strict)"("Visible"=TRUE) -> ()  [unwired: 2 in, 2 out]
                n208 = property on="Test Slider" class="Slide (strict)"("Visible"=FALSE) -> ()  [unwired: 2 in, 2 out]
              }
              frame Default {
                n209 = property on="Test Ring" class="Ring (strict)"("Visible"=FALSE) -> ()  [unwired: 2 in, 2 out]
                n210 = property on="Test Slider" class="Slide (strict)"("Visible"=FALSE) -> ()  [unwired: 2 in, 2 out]
              }
              frame "Brightness  **", "Color Level  **", "Compression  **", "FPS  **", "Sharpness  **" {
                n211 = call <vilib>:"NT Read Number.vi"("Name"=w346) -> ("Numeric"=w345:dbl)  [unwired: 9 in, 1 out]
                n212 = local write "Test Slider"(w345) -> ()
                n213 = property on="Test Slider" class="Slide (strict)"("Visible"=TRUE, "Scale.Maximum"=100.0 ("Scale.Range:Maximum")) -> ()  [unwired: 2 in, 2 out]
                n214 = property on="Test Ring" class="Ring (strict)"("Visible"=FALSE) -> ()  [unwired: 2 in, 2 out]
              }
            }
          }
        }
        n215 = property on="Progress" class="Clust (strict)"("Visible"=FALSE) -> ()  [unwired: 2 in, 2 out]
      }
      event "Test Name": Mouse Enter {
        # "Populate the ring with the list of tests"
        n216 = event-data() -> ()  [unwired: 1 in, 1 out]
        n217 = call <vilib>:"NT Read String Array.vi"("Name"="/TestMode/TestList") -> ("String Array"=w355:string[])  [unwired: 9 in, 1 out]
        n218 = Build Array (concatenate)("Select the test to run...", w355) -> (w354:string[])
        n219 = property on="Test Name" class="Ring (strict)"("Strings []"=w354) -> ()  [unwired: 2 in, 2 out]
      }
      event "Test Name": Value Change {
        w358 = FALSE ("Visible")
        # "Tell the robot the test name to run"
        n220 = event-data() -> ("NewVal"=w362:u16)  [unwired: 1 in]
        n221 = property on="Test Name" class="Ring (strict)"() -> ("Strings []"=w363:string[])  [unwired: 2 in, 2 out]
        n222 = local write "Progress"(T7 {"Test Progress"=0, "Test Progress Text"=""} ("Progress")) -> ()
        n223 = Index Array(array=w363, index=w362) -> (element=w361:string)
        n224 = call <vilib>:"NT Write String.vi"("String"=w361, "Name"="/TestMode/TestName") -> ()  [unwired: 9 in, 1 out]
        n225 = property on="Progress" class="Clust (strict)"("Visible"=TRUE) -> ()  [unwired: 2 in, 2 out]
        n226 = property on="Motor" class="Clust (strict)"("Visible"=w358) -> ()  [unwired: 2 in, 2 out]
        n227 = property on="Test Slider" class="Slide (strict)"("Visible"=w358) -> ()  [unwired: 2 in, 2 out]
        n228 = property on="On/Off" class="Bool (strict)"("Visible"=w358) -> ()  [unwired: 2 in, 2 out]
        n229 = property on="Rev/Fwd" class="Clust (strict)"("Visible"=w358) -> ()  [unwired: 2 in, 2 out]
        n230 = property on="Test Ring" class="Ring (strict)"("Visible"=w358) -> ()  [unwired: 2 in, 2 out]
      }
      event "Select Auto": Mouse Enter {
        # "Populate the combo box with the list of autonomous options"
        n231 = event-data() -> ()  [unwired: 1 in, 1 out]
        n232 = call <vilib>:"NT Read String Array.vi"("Name"="Auto List") -> ("String Array"=w365:string[])  [unwired: 9 in, 1 out]
        n233 = property on="Select Auto" class="CmbBox"("Strings[]"=w365) -> ()  [unwired: 2 in, 2 out]
      }
      event "Select Auto": Value Change {
        # "User modified the Auto Selection. Write to NT variable so robot knows."
        n234 = event-data() -> ("NewVal"=w369:string)  [unwired: 1 in]
        n235 = call <vilib>:"NT Write String.vi"("String"=w369, "Name"="Auto Selector") -> ()  [unwired: 9 in, 1 out]
      }
      event "Command Selection": Value Change {
        # "Get the params and show in table"
        n236 = event-data() -> ("NewVal"=w376:i32)  [unwired: 1 in]
        n237 = property on="Command Selection" class="MCListbox (strict)"() -> ("ItemNames"=w374:string[][])  [unwired: 2 in, 2 out]
        n238 = call <vilib>:"WPI_DashboardUpdate Command Params.vi"("NewVal"=w376, "Commands"=w374, "Param Tbl"=w375) -> ()  [unwired: 8 in, 1 out]
      }
      event "Execute Command": Value Change {
        # "Started one, Unique ID holds\nresponse"
        n239 = event-data() -> ()  [unwired: 1 in, 1 out]
        n240 = property on="Command Selection" class="MCListbox (strict)"() -> ("ItemNames"=w388:string[][])  [unwired: 2 in, 2 out]
        n241 = Index Array(array=w388, index (row)="Command Selection", index (col)=0) -> (element=w386:string)
        n242 = call <vilib>:"Invoke Commands.vi"("Command Params"="Command Params", "Function Name"=w386) -> ("Params"=w382:u8, "Started"=w381:bool)  [unwired: 7 in, 1 out]
        n243 = Array Subset(array="Command Params", length (row)=w382) -> (w383:string[][])  [unwired: 3 in]
        n244 = Select(t="Executing" ("Cmd Status"), s=w381, f="" ("Cmd Status")) -> (s? t:f=→"Cmd Status":string)
      }
      event "Command Selection": Double Click {
        n245 = event-data() -> ("Row"=w398:i32)  [unwired: 1 in]
        n246 = property on="Command Selection" class="MCListbox (strict)"() -> ("ItemNames"=w401:string[][])  [unwired: 2 in, 2 out]
        n247 = local read "Command Params"() -> (w396:string[][])
        n248 = Index Array(array=w401, index (row)=w398, index (col)=0) -> (element=w399:string)
        n249 = call <vilib>:"Invoke Commands.vi"("Command Params"=w396, "Function Name"=w399) -> ("Params"=w395:u8, "Started"=w390:bool)  [unwired: 7 in, 1 out]
        n250 = Array Subset(array=w396, length (row)=w395) -> (w394:string[][])  [unwired: 3 in]
        n251 = Select(t="Executing" ("Cmd Status"), s=w390, f="" ("Cmd Status")) -> (s? t:f=w391:string)
        n252 = local write "Cmd Status"(w391) -> ()
      }
      event "CheckList": Double Click {
        # "Shift clears all"
        # "Update symbols on the listbox"
        n253 = event-data() -> ("PlatMods.Shift"=w404:bool, "Row"=w406:i32)  [unwired: 1 in]
        n254 = case shown="True" w404 {
          tunnel: w406 -> [w410 _]
          tunnel: 1 -> [w409 _]
          frame False {
            n255 = property on="CheckList" class="LstBox (strict)"() -> ("Item Symbols"=w408:i32[])  [unwired: 2 in, 2 out]
            n256 = Replace Array Subset(array=w408, new element=w409, index=w410) -> (w407:i32[])
            n257 = property on="CheckList" class="LstBox (strict)"("Item Symbols"=w407) -> ()  [unwired: 2 in, 2 out]
          }
          frame True {
            w411 = 0 ("Top Row")
            n258 = property on="CheckList" class="LstBox (strict)"() -> ("Number of Rows"=w413:u32)  [unwired: 2 in, 2 out]
            n259 = Initialize Array(0, w413) -> (w412:i32[])
            n260 = property on="CheckList" class="LstBox (strict)"("Top Row"=w411, "Value"=w411, "Item Symbols"=w412) -> ()  [unwired: 2 in, 2 out]
          }
        }
      }
      event "CheckList": Key Down {
        # "Update symbols on the listbox\nLeft and right keys check and uncheck"
        n261 = event-data() -> ("VKey"=w418:T22)  [unwired: 1 in]
        n262 = case shown="\"Left\", \"Right\"" w418 {
          selector: w418 -> [w423 _]
          tunnel: eventvkey."Left" ("VKey") -> [w421 _]
          frame "Left", "Right" {
            n263 = Equal?(x=w421, y=w423) -> (x = y?=w422:bool)
            n264 = Select(t=0, s=w422, f=1) -> (s? t:f=w424:i32)
            n265 = property on="CheckList" class="LstBox (strict)"() -> ("Item Symbols"=w427:i32[])  [unwired: 2 in, 2 out]
            n266 = Replace Array Subset(array=w427, new element=w424, index="CheckList") -> (w426:i32[])
            n267 = property on="CheckList" class="LstBox (strict)"("Item Symbols"=w426) -> ()  [unwired: 2 in, 2 out]
          }
          frame Default {
          }
        }
      }
      event "DB Camera Config": Value Change {
        # "Show or hide the cluster of controls, store in ini file"
        n268 = event-data() -> ("NewVal"=w432:bool)  [unwired: 1 in]
        n269 = case shown="False" w432 {
          tunnel: w431 -> [w441 _]
          tunnel: [w434 w452] -> w430
          tunnel: w429 -> [w433 w452]
          frame False {
            w448 = "Camera"
            w451 = FALSE ("Visible")
            n270 = local read "Camera Settings"() -> (w440:T2)
            n271 = Index Array(array=w441) -> (element=w444:cluster{string[]})  [unwired: 1 in]
            n272 = Unbundle(w440) -> ("Frame Rate"=w439:i32, "Compression"=w438:i32, "Size"=w442:u16)
            n273 = Unbundle(w444) -> (w443:string[])
            n274 = Index Array(array=w443, index=w442) -> (element=w437:string)
            n275 = call-poly <vilib>:"Write Key.vi"("section"=w448, "value"=w437, "key"="Size", "refnum"=w433) -> ("refnum out"=w450:T20)  [unwired: 2 in, 5 out]
            n276 = call-poly <vilib>:"Write Key.vi"("section"=w448, "value"=w439, "key"="FrameRate", "refnum"=w450) -> ("refnum out"=w449:T20)  [unwired: 1 in, 6 out]
            n277 = property on="Camera Settings" class="Clust (strict)"("Visible"=w451) -> ()  [unwired: 2 in, 2 out]
            n278 = local write "DB Camera Config"(w451) -> ()
            n279 = call-poly <vilib>:"Write Key.vi"("section"=w448, "value"=w438, "key"="Compression", "refnum"=w449) -> ("refnum out"=w435:T20)  [unwired: 1 in, 6 out]
            n280 = call <vilib>:"Close Config Data.vi"("refnum"=w435) -> ("file path"=w436:path)  [unwired: 2 in, 8 out]
            n281 = call <vilib>:"Open Config Data.vi"("configuration file path"=w436) -> ("refnum"=w434:T20)  [unwired: 8 in, 2 out]
          }
          frame True {
            n282 = property on="Camera Settings" class="Clust (strict)"("Visible"=TRUE) -> ()  [unwired: 2 in, 2 out]
          }
        }
      }
      event "Camera Settings": Value Change {
        # "Update summary string when any elements of DB camera change"
        n283 = event-data() -> ("NewVal"=w466:T2)  [unwired: 1 in]
        n284 = Index Array(array=w462) -> (element=w461:cluster{string[]})  [unwired: 1 in]
        n285 = Unbundle(w466) -> ("Frame Rate"=w457:i32, "Compression"=w456:i32, "Size"=w459:u16)
        n286 = Unbundle(w461) -> (w460:string[])
        n287 = Index Array(array=w460, index=w459) -> (element=w458:string)
        n288 = Format Into String(format string="%s   %dfps   %d%%", w458, w457, w456) -> (resulting string=w463:string)  [unwired: 2 in, 1 out]
        n289 = Build Array(w463) -> (w464:string[])
        n290 = property on="DB Camera Config" class="Bool (strict)"("Strings [4]"=w464) -> ()  [unwired: 2 in, 2 out]
      }
      event "Motor.Enable": Value Change {
        # "When the test mode otor enable helper is set, update that\ntree row item's value"
        n291 = event-data() -> ("NewVal"=w473:bool)  [unwired: 1 in]
        n292 = Unbundle("Motor") -> ("Value"=w472:dbl)  [unwired: 1 out]
        n293 = Select(t=w472, s=w473, f=0.0) -> (s? t:f=w470:dbl)
        n294 = call <vilib>:"NT Write Number.vi"("Numeric"=w470, "Name"=w469) -> ()  [unwired: 9 in, 1 out]
      }
      event "Test Slider": Value Change {
        # "When the test mode slider helper is set, update that\ntree row item's value"
        n295 = event-data() -> ("NewVal"=w477:dbl)  [unwired: 1 in]
        n296 = call <vilib>:"NT Write Number.vi"("Numeric"=w477, "Name"=w478) -> ()  [unwired: 9 in, 1 out]
      }
      event "On/Off": Value Change {
        # "When the test mode on/off helper value is set, update that\ntree row item's value"
        n297 = event-data() -> ("NewVal"=w483:bool)  [unwired: 1 in]
        n298 = Boolean To (0,1)(Boolean=w483) -> (0, 1=w482:i16)
        n299 = call <vilib>:"NT Write Number.vi"("Numeric"=w482, "Name"=w481) -> ()  [unwired: 9 in, 1 out]
      }
      event "Rev/Fwd": Value Change {
        # "When the test mode helper value for relays is set, update that\ntree row item's value"
        n300 = event-data() -> ("NewVal.Forward"=w492:bool, "NewVal.Reverse"=w491:bool)  [unwired: 1 in]
        n301 = Boolean To (0,1)(Boolean=w492) -> (0, 1=w488:i16)
        n302 = Boolean To (0,1)(Boolean=w491) -> (0, 1=w490:i16)
        n303 = Negate(x=w490) -> (-x=w489:i16)
        n304 = Add(x=w488, y=w489) -> (x+y=w487:i16)
        n305 = call <vilib>:"NT Write Number.vi"("Numeric"=w487, "Name"=w486) -> ()  [unwired: 9 in, 1 out]
      }
      event "Test Ring": Value Change {
        # "When a test mode helper value is selected from the ring,\nset the tree item's variable to the string value"
        n306 = event-data() -> ("NewVal"=w497:u16)  [unwired: 1 in]
        n307 = property on="Test Ring" class="Ring (strict)"() -> ("Strings []"=w498:string[])  [unwired: 2 in, 2 out]
        n308 = Index Array(array=w498, index=w497) -> (element=w496:string)
        n309 = call <vilib>:"NT Write String.vi"("String"=w496, "Name"=w495) -> ()  [unwired: 9 in, 1 out]
      }
      event "Rec Mode": Value Change {
        # "Update globals for recording mode and path to read log from.\nClear when logging and let NetworkTables set path for vision to\nuse."
        n310 = event-data() -> ("NewVal"=w510:enum32{"Stop", "Record", "Playback"})  [unwired: 1 in]
        n311 = global write "WPI_DashboardLogging Global.vi" "Logging Filename"(path "") -> ()
        n312 = global write "WPI_DashboardLogging Global.vi" "Recording"(w510) -> ()
        n313 = case shown="\"Playback\"" w510 {
          tunnel: w509 -> [_ w512 w521]
          tunnel: [_ _ w520] -> w506
          tunnel: [_ _ w519] -> _
          tunnel: w504 -> [_ _ w517]
          tunnel: cluster{i32, i32} {-250, 170} -> [_ _ w516]
          tunnel: [_ _ T23 {"Image Size"=TRUE, "Image Type"=TRUE, "Pixel Value"=TRUE, "ROI Information"=TRUE, "Zoom Factor"=FALSE} ("Image Information Shown:All Elements")] -> w502
          tunnel: [_ _ TRUE ("Zoom Factor")] -> w501
          tunnel: w500 -> [_ _ w513]
          frame Default {
          }
          frame "Stop", "Record" {
            # "Place Window too"
            n314 = invoke class="VI" method="FP.Close"(reference=w512) -> (reference out=w511:refnum<vi>)  [unwired: 2 in, 2 out]
            n315 = invoke class="VI" method="Abort VI"(reference=w511) -> ()  [unwired: 2 in, 3 out]
          }
          frame "Playback" {
            n316 = call "Open Playback Panel.vi"("Offset"=w516, "DB VI Ref"=w517, "Playback in"=w521) -> ("Playback out"=w518:refnum<vi>)  [unwired: 8 in]
            n317 = register-events(w518, w513) -> (reference out=w520:refnum<event-registration>, error out=w519:errorcluster)  [unwired: 2 in]
          }
        }
        n318 = property on="Camera Image" class="ImageControl"("Image Information Shown"=w502, "Image Information Visible"=w501) -> ()  [unwired: 2 in, 2 out]
        n319 = call <vilib>:"WPI_DashboardNT Log FieldName Cache.vi"("Operation"=enum16{"Lookup/Add", "Index", "Clear"}."Clear") -> ()  [unwired: 8 in, 3 out]
      }
      event Panel Close {
        w523 = enum32{"Stop", "Record", "Playback"}."Stop" ("Rec Mode")
        # "Playback window has been closed, abort"
        n320 = event-data() -> ()  [unwired: 1 in, 4 out]
        n321 = local write "Rec Mode"(w523) -> ()
        n322 = global write "WPI_DashboardLogging Global.vi" "Recording"(w523) -> ()
      }
      event Panel Close {
        # "Abort playback window and ourself"
        n323 = event-data() -> ()  [unwired: 1 in, 4 out]
        n324 = invoke class="VI" method="FP.Close"(reference=w529) -> (reference out=w528:refnum<vi>)  [unwired: 2 in, 2 out]
        n325 = invoke class="VI" method="Abort VI"(reference=w528) -> (error out=w527:errorcluster)  [unwired: 2 in, 2 out]
        n326 = invoke class="VI" method="Abort VI"(error in=w527) -> ()  [unwired: 2 in, 3 out]
      }
      event User Event {
        n327 = event-data() -> ("IDs"=w537:cluster{"RPC field ID":u16, "Unique ID":u16}, "String"=w536:string)  [unwired: 1 in]
        n328 = Bundle("IDs"=w537, "String"=w536) -> (w535:T9)  [unwired: 1 in]
        n329 = call <vilib>:"Retrieve RPC Response.vi"("RPC Response"=w535) -> ("Output"=w532:string[][])  [unwired: 10 in]
        n330 = Build Array (concatenate)(w530, w532) -> (w531:string[][])
        n331 = local write "Command Params"(w531) -> ()
        n332 = local write "Cmd Status"("" ("Cmd Status")) -> ()
      }
      event "Vision": Value Change {
        # "Enable/Disable Compression slider.\nHW USB is hard-coded into the camera"
        n333 = event-data() -> ("NewVal"=w544:u16)  [unwired: 1 in]
        n334 = Equal?(x=w544, y=u32 2 ("milliseconds to wait")) -> (x = y?=w542:bool)
        n335 = Select(t=T24."Disabled and Grayed Out" ("Disabled"), s=w542, f=T24."Enabled" ("Disabled")) -> (s? t:f=w539:T24)
        n336 = property on="Compression" class="Slide (strict)"("DisabledEnum"=w539) -> ()  [unwired: 2 in, 2 out]
      }
      event "Tree": Double Click {
        n337 = event-data() -> ("PlatMods"=w549:T27, "Tag"=w548:string)  [unwired: 1 in]
        n338 = Unbundle(w549) -> ("Shift"=w547:bool)  [unwired: 4 out]
        n339 = Not(x=w547) -> (.not. x?=w546:bool)
        n340 = call <vilib>:"NT Update Persistence.vi"("Persistence"=w546, "Name"=w548) -> ()  [unwired: 9 in, 1 out]
      }
    }
  }
  n341 = while {
    tunnel: w47 -> [w553]
    i -> [w556]
    stop <- FALSE stop-if-true
    n342 = Wait (ms)(milliseconds to wait=u32 100) -> ()  [unwired: 1 out]
    n343 = case shown="\"Playback\"" "Rec Mode" {
      tunnel: w556 -> [_ _ w571]
      tunnel: [u32 2829099 ("Base Color") u32 11141120 ("Target Color") w560] -> w552
      frame "Stop", Default {
        # "Reset the color, extra updates don't cost much"
      }
      frame "Record" {
      }
      frame "Playback" {
        # "Playback"
        n344 = Quotient & Remainder(x=w571, y=u32 50 ("milliseconds to wait")) -> (x-y*floor(x/y)=w567:u32)  [unwired: 1 out]
        n345 = Divide(x=w567, y=u32 50 ("milliseconds to wait")) -> (x/y=w564:dbl)
        n346 = Multiply(x=6.283185307179586, y=w564) -> (x*y=w569:dbl)
        n347 = Sine(x=w569) -> (sin(x)=w568:dbl)
        n348 = Absolute Value(x=w568) -> (abs(x)=w561:dbl)
        n349 = call "Interpolate RGB Color.vi"("Proportion"=w561, "Target Color"=u32 30976, "Base Color"=u32 2829099) -> ("Result Color"=w560:u32)  [unwired: 8 in]
      }
    }
    n350 = property class="Pane"(reference=w553, "PaneColor"=w552) -> ()  [unwired: 1 in, 2 out]
  }
  n351 = local write "Dashboard Tab"(T1."Drive" ("Dashboard Tab")) -> ()
  n352 = property on="On/Off" class="Bool (strict)"("Visible"=w15) -> ()  [unwired: 2 in, 2 out]
  n353 = property on="Motor" class="Clust (strict)"("Visible"=w15) -> ()  [unwired: 2 in, 2 out]
  n354 = property on="Progress" class="Clust (strict)"("Visible"=w15) -> ()  [unwired: 2 in, 2 out]
  n355 = property on="Test Ring" class="Ring (strict)"("Visible"=w15) -> ()  [unwired: 2 in, 2 out]
  n356 = property on="Rev/Fwd" class="Clust (strict)"("Visible"=w15) -> ()  [unwired: 2 in, 2 out]
  n357 = property on="Camera Settings" class="Clust (strict)"("Visible"=w15) -> ()  [unwired: 2 in, 2 out]
  n358 = while {
    tunnel: u16 1741 ("timeout ms (25000)") -> [w573]
    stop <- FALSE stop-if-true
    n359 = TCP Create Listener(10:w573) -> (0:w572:errorcluster, 3:w574:refnum<k5>)  [unwired: 4 in, 1 out]
    n360 = case shown="No Error" w572 {
      selector: w572 -> [w576 _]
      tunnel: w574 -> [w577 _]
      frame No Error {
        n361 = while {
          tunnel: w577 -> [w580]
          tunnel: w576 -> [w579]
          stop <- FALSE stop-if-true
          n362 = TCP Wait On Listener(8:w579, 11:w580) -> (0:w581:errorcluster, 4:w582:refnum<k5>)  [unwired: 2 in, 3 out]
          n363 = local write "TCP"(w582) -> ()
          n364 = case shown="No Error" w581 {
            frame No Error {
            }
            frame Error {
              n365 = Wait (ms)(milliseconds to wait=u32 1000) -> ()  [unwired: 1 out]
            }
          }
        }
      }
      frame Error {
        n366 = Wait (ms)(milliseconds to wait=u32 1000) -> ()  [unwired: 1 out]
      }
    }
  }
  n367 = local write "DB Camera Config"(w15) -> ()
  n368 = local write "Command Params"(string[][] [] ("Command Params")) -> ()
  n369 = global write "WPI_DashboardLogging Global.vi" "Recording"(w41) -> ()
  n370 = local write "Command Selection"(u16 0 ("milliseconds to wait")) -> ()
  n371 = local write "Rec Mode"(w41) -> ()
